vi "3a - Write global.vi"() -> ()   [LabVIEW 2010]
uses:
  My Globals.vi
panel:
  in  "stop":bool
  out "Chart 2":dbl(graph)
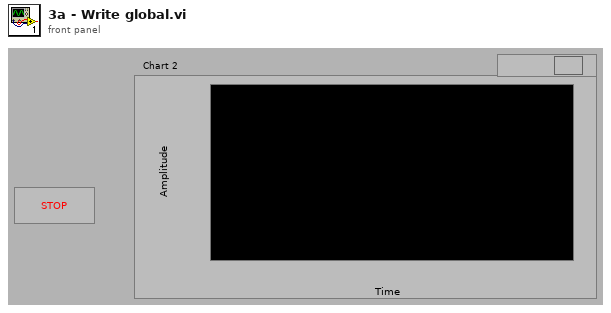
[diagram p1: front panel]
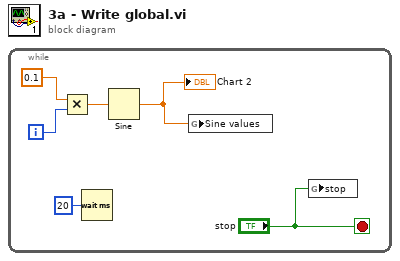
[diagram p0: block diagram]
diagram:
  n1 = while {
    i -> [w4]
    stop <- "stop" stop-if-true
    n2 = Multiply(x=0.1, y=w4) -> (x*y=w3:dbl)
    n3 = Wait (ms)(milliseconds to wait=u32 20) -> ()  [unwired: 1 out]
    n4 = Sine(x=w3) -> (sin(x)=w1:dbl)
    "Chart 2" <- w1
    n5 = global write "My Globals.vi" "Sine values"(w1) -> ()
    n6 = global write "My Globals.vi" "stop"("stop") -> ()
  }
